vi "MonitorGlobals.vi"() -> ()   [LabVIEW 2015]
panel:
  out "MonitorInitDone":bool
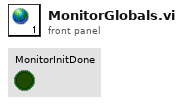
[diagram p1: front panel]
diagram:
